vi "Create AFDX MAC (Dest).vi"(11 "VL Id":u16) -> (3 "MAC-src":u8[](array[numeric]) format="%02x")   [LabVIEW 2020, in "EthFrameManagement.lvlib"]
uses:
  EthFrameManagement.lvlib
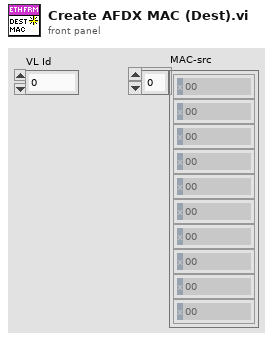
[diagram p1: front panel]
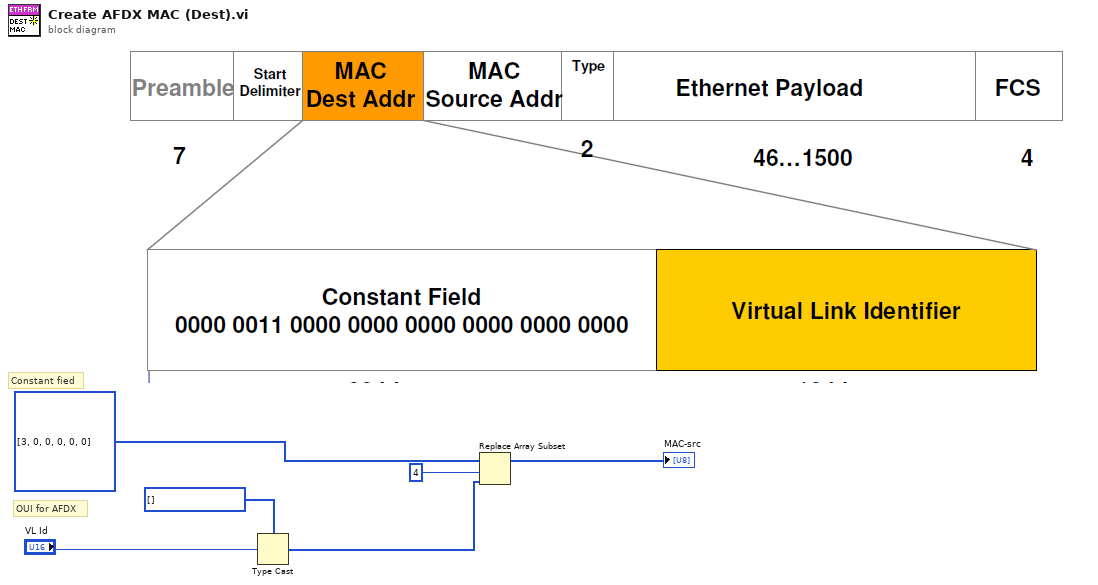
[diagram p0: block diagram]
diagram:
  # "OUI for AFDX"
  # "Constant fied"
  n1 = Type Cast(type=u8[] [] ("MAC-src"), x="VL Id") -> (*(type *) &x=w1:u8[])
  n2 = Replace Array Subset(array=u8[] [3, 0, 0, 0, 0, 0] ("MAC-src"), new element=w1, index=4) -> (→"MAC-src":u8[])
